vi "RANSACRegressor.vi"(8 "error in":errorcluster) -> (0 "error out":errorcluster, 3 "out":refnum<class "RANSACRegressor.lvclass">)   [LabVIEW 2020]
doc: "RANSAC (RANdom SAmple Consensus) algorithm.\n\n RANSAC is an iterative algorithm for the robust estimation of parameters\n from a subset of inliers from the complete data set.\n\n Read more in the :ref:`User Guide <ransac_regression>`.\n\n Parameters\n ----------\n base_estimator : object, default=None\n Base estimator object which implements the following methods:\n\n * `fit(X, y)`: Fit model to given training data and target values.\n * `score(X, y)`: Returns the mean accuracy on the given test data,\n which is used for the stop criterion defined by `stop_score`.\n Additionally, the score is used to decide which of two equally\n large consensus sets is chosen as the better one.\n * `predict(X)`: Returns predicted values using the linear model,\n which is used to compute residual error using loss function.\n\n If `base_estimator` is None, then\n :class:`~sklearn.linear_model.LinearRegression` is used for\n target values of dtype float.\n\n Note that the current implementation only supports regression\n estimators.\n\n min_samples : int (>= 1) or float ([0, 1]), default=None\n Minimum number of samples chosen randomly from original data. Treated\n as an absolute number of samples for `min_samples >= 1`, treated as a\n relative number `ceil(min_samples * X.shape[0]`) for\n `min_samples < 1`. This is typically chosen as the minimal number of\n samples necessary to estimate the given `base_estimator`. By default a\n ``sklearn.linear_model.LinearRegression()`` estimator is assumed and\n `min_samples` is chosen as ``X.shape[1] + 1``.\n\n residual_threshold : float, default=None\n Maximum residual for a data sample to be classified as an inlier.\n By default the threshold is chosen as the MAD (median absolute\n deviation) of the target values `y`.\n\n is_data_valid : callable, default=None\n This function is called with the randomly selected data before the\n model is fitted to it: `is_data_valid(X, y)`. If its return value is\n False the current randomly chosen sub-sample is skipped.\n\n is_model_valid : callable, default=None\n This function is called with the estimated model and the randomly\n selected data: `is_model_valid(model, X, y)`. If its return value is\n False the current randomly chosen sub-sample is skipped.\n Rejecting samples with this function is computationally costlier than\n with `is_data_valid`. `is_model_valid` should therefore only be used if\n the estimated model is needed for making the rejection decision.\n\n max_trials : int, default=100\n Maximum number of iterations for random sample selection.\n\n max_skips : int, default=np.inf\n Maximum number of iterations that can be skipped due to finding zero\n inliers or invalid data defined by ``is_data_valid`` or invalid models\n defined by ``is_model_valid``.\n\n .. versionadded:: 0.19\n\n stop_n_inliers : int, default=np.inf\n Stop iteration if at least this number of inliers are found.\n\n stop_score : float, default=np.inf\n Stop iteration if score is greater equal than this threshold.\n\n stop_probability : float in range [0, 1], default=0.99\n RANSAC iteration stops if at least one outlier-free set of the training\n data is sampled in RANSAC. This requires to generate at least N\n samples (iterations)::\n\n N >= log(1 - probability) / log(1 - e**m)\n\n where the probability (confidence) is typically set to high value such\n as 0.99 (the default) and e is the current fraction of inliers w.r.t.\n the total number of samples.\n\n loss : string, callable, default='absolute_loss'\n String inputs, \"absolute_loss\" and \"squared_loss\" are supported which\n find the absolute loss and squared loss per sample\n respectively.\n\n If ``loss`` is a callable, then it should be a function that takes\n two arrays as inputs, the true and predicted value and returns a 1-D\n array with the i-th value of the array corresponding to the loss\n on ``X[i]``.\n\n If the loss on a sample is greater than the ``residual_threshold``,\n then this sample is classified as an outlier.\n\n .. versionadded:: 0.18\n\n random_state : int, RandomState instance, default=None\n The generator used to initialize the centers.\n Pass an int for reproducible output across multiple function calls.\n See :term:`Glossary <random_state>`.\n\n Attributes\n ----------\n estimator_ : object\n Best fitted model (copy of the `base_estimator` object).\n\n n_trials_ : int\n Number of random selection trials until one of the stop criteria is\n met. It is always ``<= max_trials``.\n\n inlier_mask_ : bool array of shape [n_samples]\n Boolean mask of inliers classified as ``True``.\n\n n_skips_no_inliers_ : int\n Number of iterations skipped due to finding zero inliers.\n\n .. versionadded:: 0.19\n\n n_skips_invalid_data_ : int\n Number of iterations skipped due to invalid data defined by\n ``is_data_valid``.\n\n .. versionadded:: 0.19\n\n n_skips_invalid_model_ : int\n Number of iterations skipped due to an invalid model defined by\n ``is_model_valid``.\n\n .. versionadded:: 0.19\n\n \nAvailable methods:\nGet Attributes\nGet Params\nSet Params"
uses:
  RANSACRegressor.lvclass
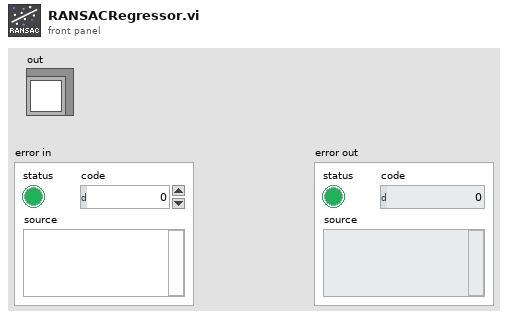
[diagram p1: front panel]
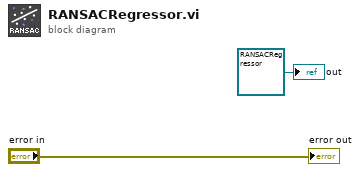
[diagram p0: block diagram]
diagram:
  "out" <- refnum<class "RANSACRegressor.lvclass"> refnum ("model")
  "error out" <- "error in"
